vi "Pololu Find Alias.vi"(8 "error in":errorcluster, 10 "PID":string, 11 "VID":string) -> (0 "error out":errorcluster, 3 "Alias":string)   [LabVIEW 2018]
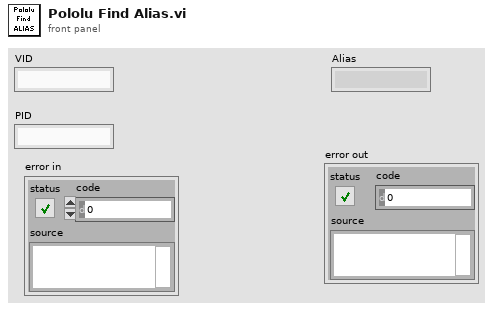
[diagram p1: front panel]
types:
  T1 = typedef "VISA.Device Info.ctl" = cluster{"Match":i32, "Alias":string, "Description":string, "Available":bool, "PID":string, "VID":string}
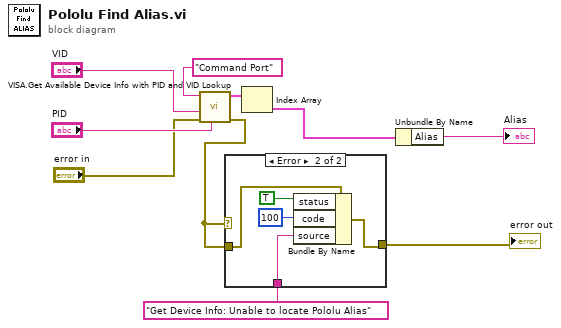
[diagram p0: block diagram]
diagram:
  n1 = call "VISA.Get Available Device Info with PID and VID Lookup.vi"("PID"="PID", "error in"="error in", "VID"="VID", "Alias Contains"="Command Port") -> ("error out"=w9:errorcluster, "Devices"=w5:T1[])  [unwired: 5 in, 1 out]
  n2 = case shown="Error" w9 {
    tunnel: [w11 w12] -> w10
    tunnel: "Get Device Info: Unable to locate Pololu Alias" ("Description") -> [_ w13]
    tunnel: w9 -> [w11 w16]
    frame No Error {
    }
    frame Error {
      n3 = Bundle By Name(cluster=w16, "status"=TRUE ("Append Details"), "code"=100 ("Code(0 = no change)"), "source"=w13) -> (w12:errorcluster)
    }
  }
  "error out" <- w10
  n4 = Index Array(array=w5) -> (element=w6:T1)  [unwired: 1 in]
  n5 = Unbundle By Name(w6) -> ("Alias"=→"Alias":string)
